vi "conveyor-machine-rpm.vi"(2 "speed in":i32(listbox), 3 "Temperature in":dbl(slide) scale=0.0..100.0) -> (0 "rpm out":dbl(knob) scale=0.0..10.0, 1 "Temperature out":dbl(slide) scale=0.0..100.0)   [LabVIEW 2026]
uses:
  <vilib>/numeric/Random Number (Range) DBL.vi
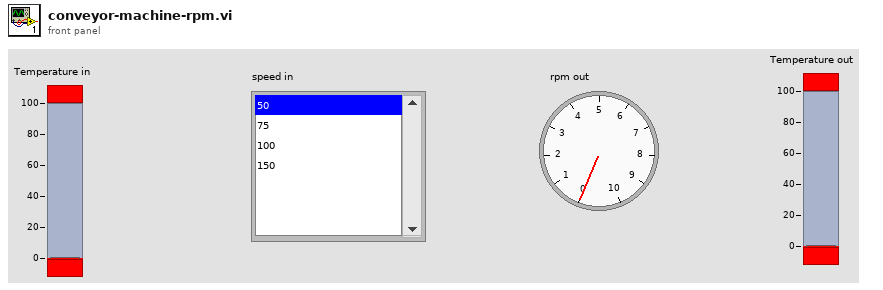
[diagram p1: front panel]
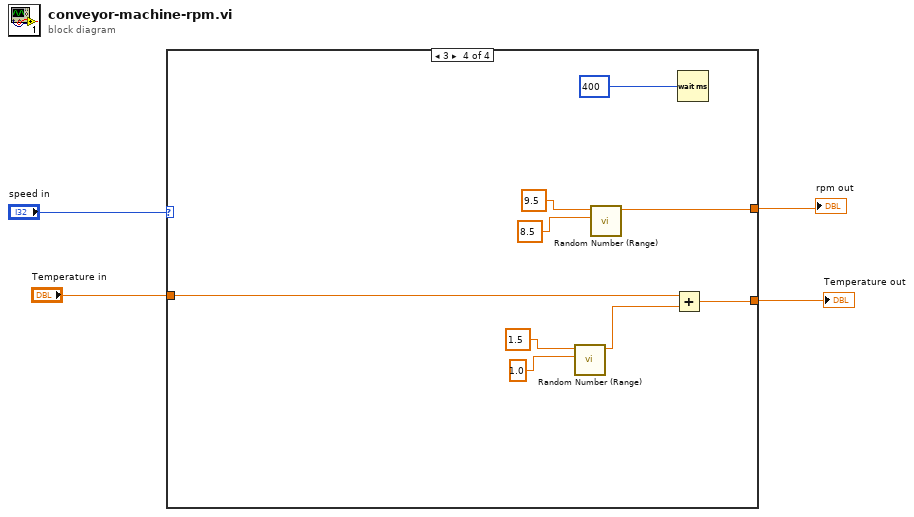
[diagram p0: block diagram]
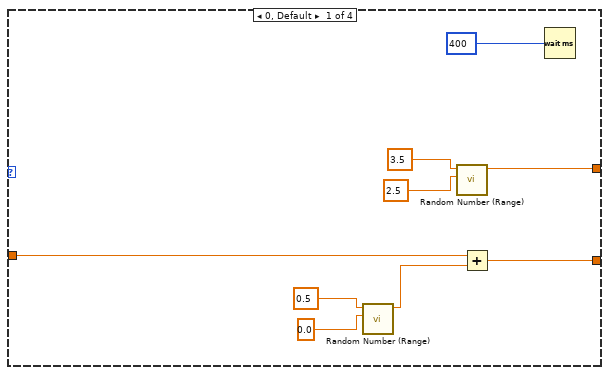
[diagram p2: hidden frame]
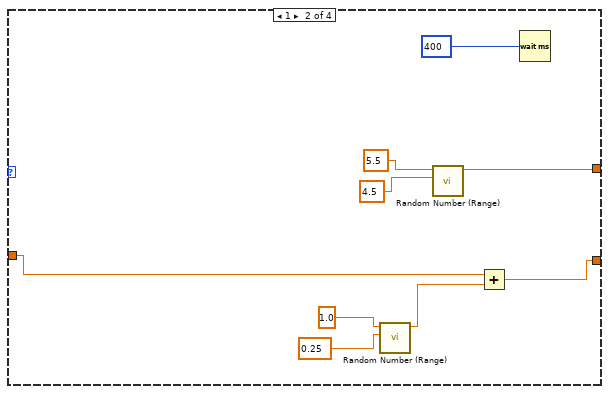
[diagram p3: hidden frame]
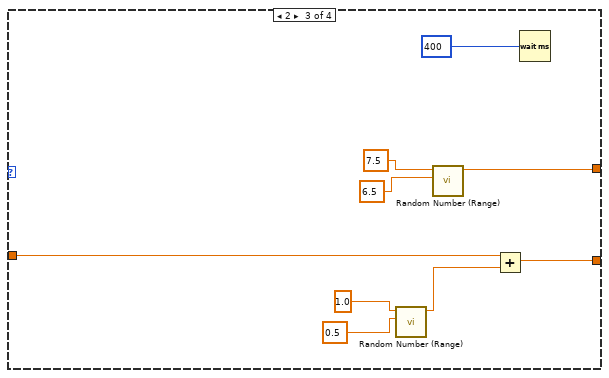
[diagram p4: hidden frame]
diagram:
  n1 = case shown="3" "speed in" {
    tunnel: [w10 w19 w28 w37] -> w3
    tunnel: [w7 w15 w24 w33] -> w2
    tunnel: "Temperature in" -> [w6 w14 w23 w32]
    frame 0, Default {
      n2 = call-poly <vilib>:"Random Number (Range).vi"("lower bound (0)"=0.0, "upper bound (100)"=0.5) -> ("number"=w5:dbl)  [unwired: 9 in]
      n3 = call-poly <vilib>:"Random Number (Range).vi"("lower bound (0)"=2.5, "upper bound (100)"=3.5) -> ("number"=w10:dbl)  [unwired: 9 in]
      n4 = Add(x=w6, y=w5) -> (x+y=w7:dbl)
      n5 = Wait (ms)(milliseconds to wait=u32 400) -> ()  [unwired: 1 out]
    }
    frame 1 {
      n6 = call-poly <vilib>:"Random Number (Range).vi"("lower bound (0)"=0.25, "upper bound (100)"=1.0) -> ("number"=w16:dbl)  [unwired: 9 in]
      n7 = call-poly <vilib>:"Random Number (Range).vi"("lower bound (0)"=4.5, "upper bound (100)"=5.5) -> ("number"=w19:dbl)  [unwired: 9 in]
      n8 = Add(x=w14, y=w16) -> (x+y=w15:dbl)
      n9 = Wait (ms)(milliseconds to wait=u32 400) -> ()  [unwired: 1 out]
    }
    frame 2 {
      n10 = call-poly <vilib>:"Random Number (Range).vi"("lower bound (0)"=0.5, "upper bound (100)"=1.0) -> ("number"=w25:dbl)  [unwired: 9 in]
      n11 = call-poly <vilib>:"Random Number (Range).vi"("lower bound (0)"=6.5, "upper bound (100)"=7.5) -> ("number"=w28:dbl)  [unwired: 9 in]
      n12 = Add(x=w23, y=w25) -> (x+y=w24:dbl)
      n13 = Wait (ms)(milliseconds to wait=u32 400) -> ()  [unwired: 1 out]
    }
    frame 3 {
      n14 = call-poly <vilib>:"Random Number (Range).vi"("lower bound (0)"=1.0, "upper bound (100)"=1.5) -> ("number"=w36:dbl)  [unwired: 9 in]
      n15 = call-poly <vilib>:"Random Number (Range).vi"("lower bound (0)"=8.5, "upper bound (100)"=9.5) -> ("number"=w37:dbl)  [unwired: 9 in]
      n16 = Add(x=w32, y=w36) -> (x+y=w33:dbl)
      n17 = Wait (ms)(milliseconds to wait=u32 400) -> ()  [unwired: 1 out]
    }
  }
  "rpm out" <- w3
  "Temperature out" <- w2
